vi "remove consecutive duplicates.vi"(10 "Array in":string[](array[string])) -> (2 "Array out":string[](array[string]))   [LabVIEW 2020]
doc: "This VI removes any consecutive duplicates from a string array."
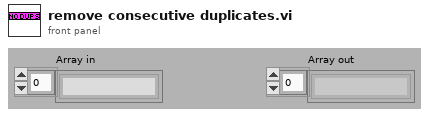
[diagram p1: front panel]
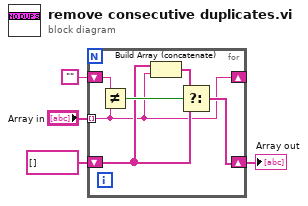
[diagram p0: block diagram]
diagram:
  n1 = for {
    tunnel: "Array in" -> [w5] mode=indexing
    shift-right: [w5] -> _
    shift-left: "" -> [w10]
    shift-right: [w6] -> w4
    shift-left: string[] [] -> [w7]
    n2 = Not Equal?(x=w10, y=w5) -> (x != y?=w9:bool)
    n3 = Build Array (concatenate)(w7, w5) -> (w8:string[])
    n4 = Select(t=w8, s=w9, f=w7) -> (s? t:f=w6:string[])
  }
  "Array out" <- w4
